vi "tester.vi"() -> ()   [LabVIEW 2012]
panel:
  in  "dx":i32=1
  out "appended array":dbl[][](array[numeric])
  out "(Xo = 10, dX = 2, Y) Multi Plot 2":cluster{"xo":i32, "dx":i32, dbl[][]}(graph)
  in  "9213 Config":T1={"Sample Rate [Hz]"=100.0, "Samples/Ch"=1, "Ch Used"=1, "Rolling Average"=1, "HI/LO Trim [%]"=1.0, "Sample Timing Engine"=2} {"Ch Used" min=1 max=16 step=1; "Sample Timing Engine" max=2; "Sample Rate [Hz]" min=0.0001 max=100.0 format="%#_6p"; "Samples/Ch" min=1 step=1; "Rolling Average" min=1 step=1; "HI/LO Trim [%]" min=1.0 max=99.0}
  out "Measurements":dbl[](array[numeric])=[-5.992573762181492, -5.997989953152922, -5.993374507791335, -6.01505502545452, -5.993954720178463, -5.998898340010818, -5.994243513683498, -6.001704887940654, -5.992164200481336, -5.997039559969114, -5.99175726418588, -6.014566701819755, -5.991988298982826, -5.998748692473846, -5.9949628720597365, -6.004621702529348] format="%.2f"
  out "Numeric":i32
  out "9213 Error":errorcluster
  in  "9213 Name":tag="9213"
  in  "stop":bool
  out "Graph":cluster{dbl, "dx":i32, dbl[][]}(graph)
  # "9213 Configuration"
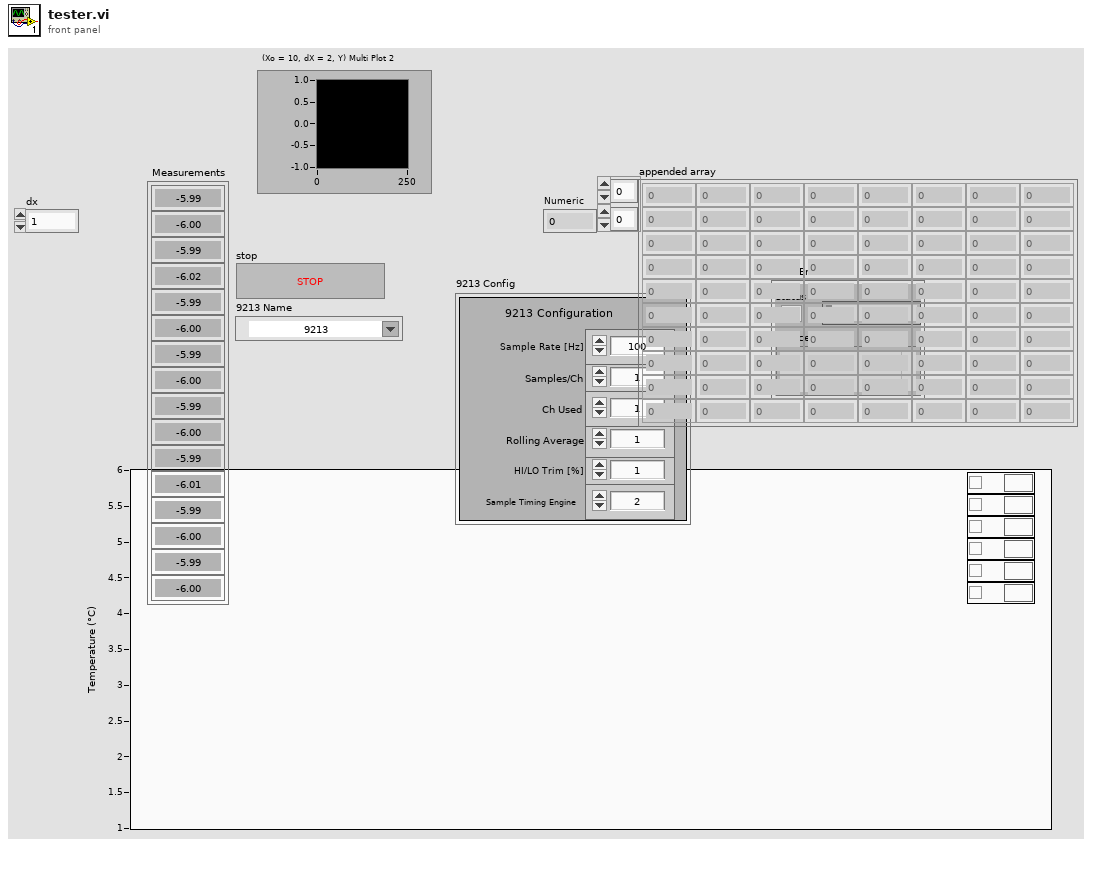
[diagram p1: front panel]
types:
  T1 = cluster{"Sample Rate [Hz]":dbl, "Samples/Ch":i32, "Ch Used":i32, "Rolling Average":i32, "HI/LO Trim [%]":dbl, "Sample Timing Engine":u32}
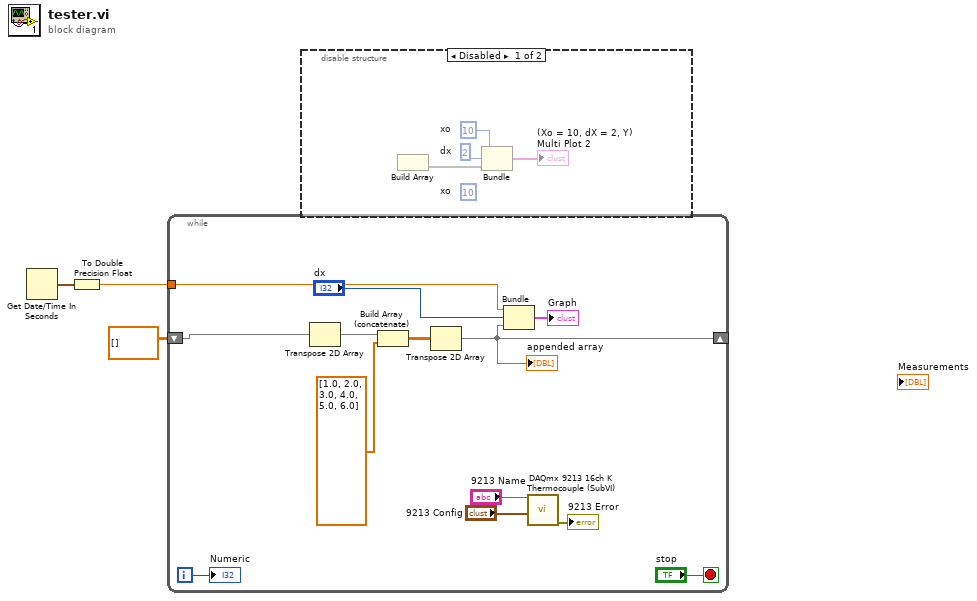
[diagram p0: block diagram]
diagram:
  n1 = Get Date/Time In Seconds() -> (seconds since 1Jan1904=w3:timestamp)
  n2 = To Double Precision Float(number=w3) -> (double precision float=w2:dbl)
  n3 = while {
    tunnel: w2 -> [w12]
    shift-right: [w5] -> _
    shift-left: dbl[][] [] -> [w6]
    i -> [w15]
    stop <- "stop" stop-if-true
    n4 = Transpose 2D Array(2D array=w6) -> (transposed array=w4:dbl[][])
    n5 = Build Array (concatenate)(w4, dbl[] [1.0, 2.0, 3.0, 4.0, 5.0, 6.0]) -> (w7:dbl[][])
    n6 = Transpose 2D Array(2D array=w7) -> (transposed array=w5:dbl[][])
    "appended array" <- w5
    n7 = Bundle(w12, "dx"="dx", w5) -> (→"Graph":cluster{dbl, "dx":i32, dbl[][]})  [unwired: 1 in]
    n8 = call "DAQmx 9213 16ch K Thermocouple (SubVI).vi"("9213 Name"="9213 Name", "9213 Config"="9213 Config") -> ("9213 Error"=→"9213 Error":errorcluster)  [unwired: 12 in, 1 out]
    "Numeric" <- w15
  }
  n9 = disable-structure shown="Disabled" {
    frame Disabled {
      (unwired) 10  # xo
      w19 = 2  # dx
      w18 = 10  # xo
      n10 = Build Array() -> (w20:void[])  [unwired: 2 in]
      n11 = Bundle("xo"=w18, "dx"=w19, w20) -> (→"(Xo = 10, dX = 2, Y) Multi Plot 2":cluster{"xo":i32, "dx":i32, void[]})  [unwired: 1 in]
    }
    frame Enabled {
    }
  }
